vi "ParseByComma.vi"(11 "String":string) -> (2 "SecondParseValue":string, 3 "FirstParseValue":string, 5 "AllParsedValue":string[](array[string]))   [LabVIEW 2018, in "Test.lvclass"]
doc: "Transforms a string control into an array of strings using a comma delimited key."
uses:
  Test.lvclass
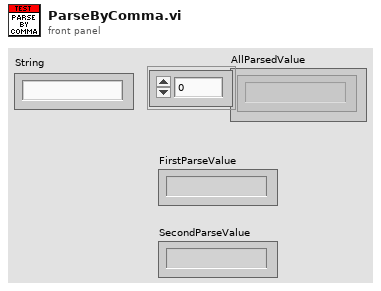
[diagram p1: front panel]
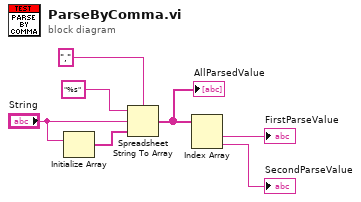
[diagram p0: block diagram]
diagram:
  n1 = Initialize Array("String") -> (w6:string[])  [unwired: 1 in]
  n2 = Spreadsheet String To Array(delimiter (Tab)=",", format string="%s", spreadsheet string="String", array type (2D Dbl)=w6) -> (array=w4:string[])
  "AllParsedValue" <- w4
  n3 = Index Array(array=w4) -> (element #1=→"FirstParseValue":string, element #2=→"SecondParseValue":string)  [unwired: 2 in]
